vi "Create_column_headers.vi"(1 "ADAM Titles":string[](array[string]), 3 "ADAM Comments":string[](array[string]), 4 "Additional Channels":string[](array[string])) -> (5 "Column headers":string[](array[string]), 6 "Header Comments":string[](array[string]), 7 "No of stats columns":i32[](array[numeric]))   [LabVIEW 2010]
uses:
  Globals/Meas_global.vi
  Globals/Dynamic_call_global.ph.vi
  Globals/LDA_meas_global_1.vi
  Acquisition/PWA/PWAtasksGLOBAL.vi
  Globals/Preference_global.vi
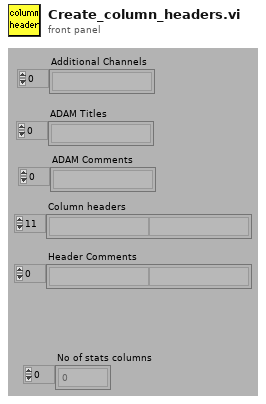
[diagram p1: front panel]
types:
  T1 = typedef "PWA_Data.ctl" = enum16{"No PWA Data", "One Ch PWA"}
  T2 = typedef "Server_Comms.ctl" = enum16{"Server Link Healthy", "Do Not Link To Server"}
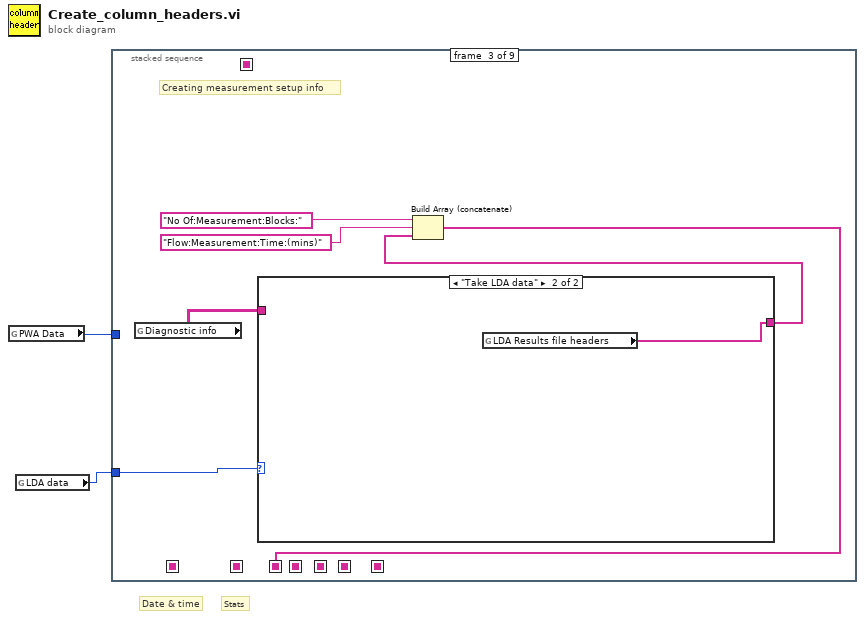
[diagram p0: block diagram]
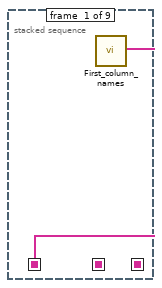
[diagram p2: hidden frame]
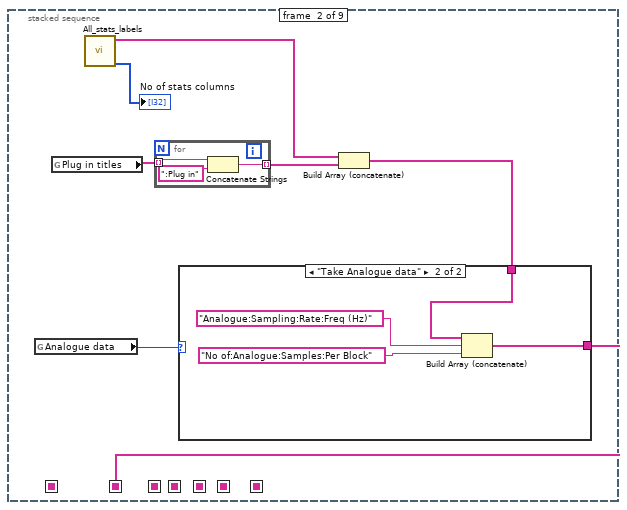
[diagram p3: hidden frame]
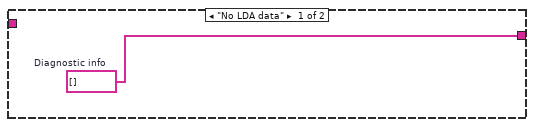
[diagram p5: hidden frame]
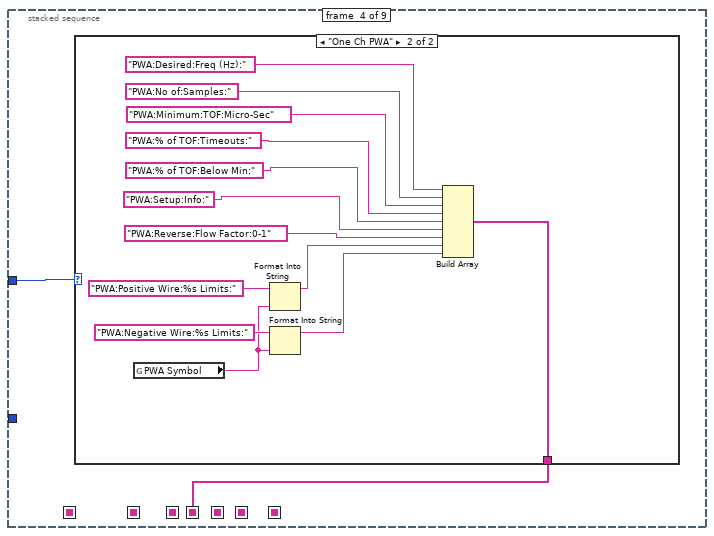
[diagram p6: hidden frame]
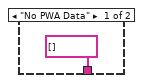
[diagram p7: hidden frame]
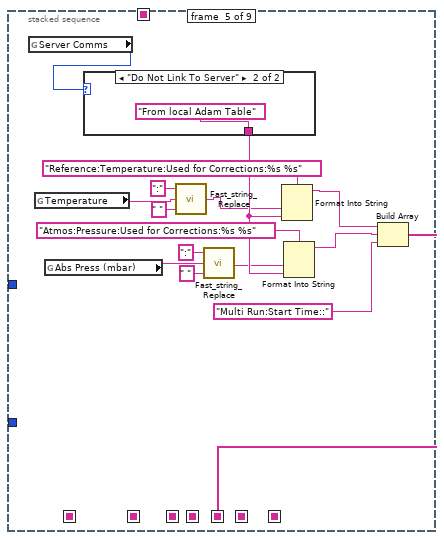
[diagram p8: hidden frame]
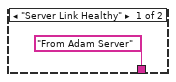
[diagram p9: hidden frame]
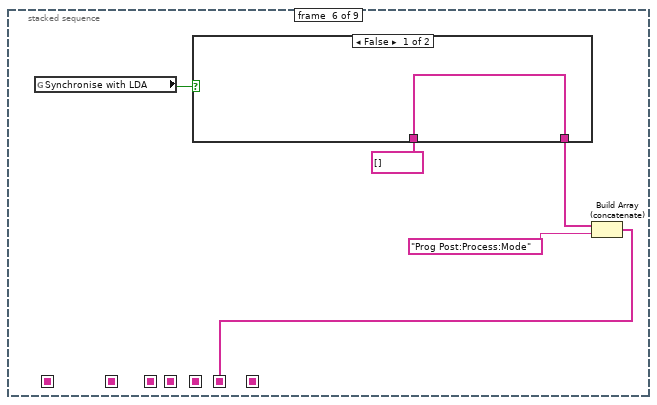
[diagram p10: hidden frame]
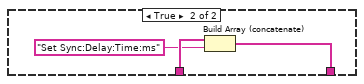
[diagram p11: hidden frame]
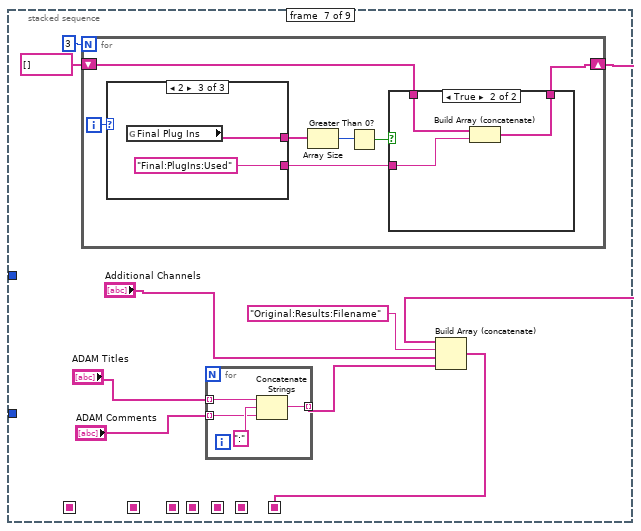
[diagram p12: hidden frame]
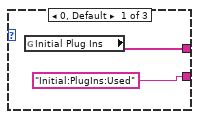
[diagram p14: hidden frame]
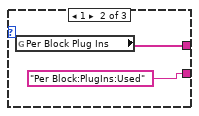
[diagram p15: hidden frame]
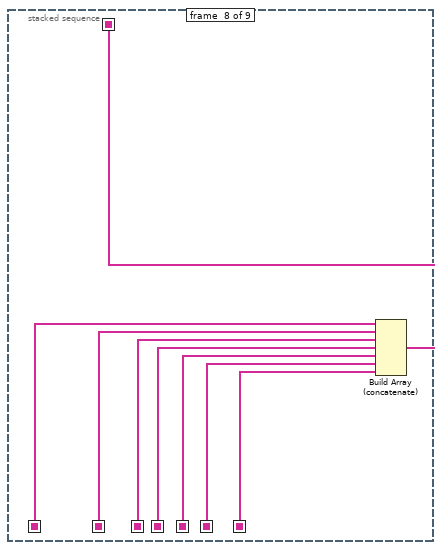
[diagram p16: hidden frame]
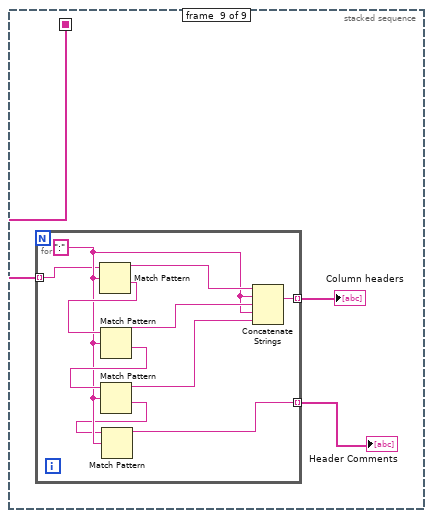
[diagram p17: hidden frame]
diagram:
  # "Stats"
  # "Date & time"
  n1 = global read "Meas_global.vi" "PWA Data"() -> (w1:T1)
  n2 = global read "Meas_global.vi" "LDA data"() -> (w2:enum16{"No LDA data", "Take LDA data"})
  n3 = stacked-sequence {
    seq-local: [_ w4 _ _ _ _ _ _ _] -> [_ _ _ _ _ _ _ w106 _]
    seq-local: [w3 _ _ _ _ _ _ _ _] -> [_ _ _ _ _ _ _ w107 _]
    seq-local: [_ _ w22 _ _ _ _ _ _] -> [_ _ _ _ _ _ _ w105 _]
    seq-local: [_ _ _ _ _ _ w71 _ _] -> [_ _ _ _ _ _ _ w101 _]
    seq-local: [_ _ _ _ w44 _ _ _ _] -> [_ _ _ _ _ _ _ w103 _]
    seq-local: [_ _ _ _ _ _ _ w104 _] -> [_ _ _ _ _ _ _ _ w109]
    seq-local: [_ _ _ _ _ w62 _ _ _] -> [_ _ _ _ _ _ _ w102 _]
    seq-local: [_ _ _ w27 _ _ _ _ _] -> [_ _ _ _ _ _ _ w100 _]
    tunnel: w2 -> [_ _ w20 _ _ _ _ _ _]
    tunnel: w1 -> [_ _ _ w28 _ _ _ _ _]
    frame #0 {
      n4 = call "First_column_names.vi"() -> ("Array"=w3:string[])
    }
    frame #1 {
      n5 = global read "Meas_global.vi" "Analogue data"() -> (w6:enum16{"No Analogue data", "Take Analogue data"})
      n6 = global read "Dynamic_call_global.ph.vi" "Plug in titles"() -> (w9:string[])
      n7 = call "All_stats_labels.vi"() -> ("No of stats columns"=→"No of stats columns":i32[], "Stats labels"=w8:string[])  [unwired: 6 out]
      n8 = for {
        tunnel: w9 -> [w17] mode=indexing
        tunnel: [w18] -> w7 mode=indexing
        n9 = Concatenate Strings(w17, ":Plug in" ("Substring")) -> (w18:string)
      }
      n10 = Build Array (concatenate)(w8, w7) -> (w5:string[])
      n11 = case shown="\"Take Analogue data\"" w6 {
        tunnel: w5 -> [w11 w13]
        tunnel: [w11 w12] -> w4
        frame "No Analogue data" {
        }
        frame "Take Analogue data" {
          n12 = Build Array (concatenate)(w13, "Analogue:Sampling:Rate:Freq (Hz)", "No of:Analogue:Samples:Per Block") -> (w12:string[])
        }
      }
    }
    frame #2 {
      # "Creating measurement setup info"
      n13 = global read "Meas_global.vi" "Diagnostic info"() -> (w21:string[][])
      n14 = case shown="\"Take LDA data\"" w20 {
        tunnel: w21 -> [_ _]
        tunnel: [w25 w26] -> w19
        frame "No LDA data" {
          w25 = string[] []  # Diagnostic info
        }
        frame "Take LDA data" {
          n15 = global read "LDA_meas_global_1.vi" "LDA Results file headers"() -> (w26:string[])
        }
      }
      n16 = Build Array (concatenate)("No Of:Measurement:Blocks:", "Flow:Measurement:Time:(mins)", w19) -> (w22:string[])
    }
    frame #3 {
      n17 = case shown="\"One Ch PWA\"" w28 {
        tunnel: [string[] [] w32] -> w27
        frame "No PWA Data" {
        }
        frame "One Ch PWA" {
          n18 = global read "PWAtasksGLOBAL.vi" "PWA Symbol"() -> (w40:string)
          n19 = Format Into String(format string="PWA:Positive Wire:%s Limits:", w40) -> (resulting string=w34:string)  [unwired: 2 in, 1 out]
          n20 = Format Into String(format string="PWA:Negative Wire:%s Limits:", w40) -> (resulting string=w33:string)  [unwired: 2 in, 1 out]
          n21 = Build Array("PWA:Desired:Freq (Hz):", "PWA:No of:Samples:", "PWA:Minimum:TOF:Micro-Sec", "PWA:% of TOF:Timeouts:", "PWA:% of TOF:Below Min:", "PWA:Setup:Info:", "PWA:Reverse:Flow Factor:0-1", w34, w33) -> (w32:string[])
        }
      }
    }
    frame #4 {
      n22 = global read "Preference_global.vi" "Server Comms"() -> (w58:T2)
      n23 = global read "Preference_global.vi" "Temperature"() -> (w50:string)
      n24 = global read "Preference_global.vi" "Abs Press (mbar)"() -> (w46:string)
      n25 = case shown="\"Do Not Link To Server\"" w58 {
        tunnel: ["From Adam Server" "From local Adam Table"] -> w53
        frame "Server Link Healthy" {
        }
        frame "Do Not Link To Server" {
        }
      }
      n26 = call "Fast_string_Replace.vi"("Replace match with:"=" ", "Input String"=w50, "regular expression"=":") -> ("Output String"=w49:string)  [unwired: 2 out]
      n27 = call "Fast_string_Replace.vi"("Replace match with:"=" ", "Input String"=w46, "regular expression"=":") -> ("Output String"=w45:string)  [unwired: 2 out]
      n28 = Format Into String(format string="Reference:Temperature:Used for Corrections:%s %s", w49, w53) -> (resulting string=w56:string)  [unwired: 2 in, 1 out]
      n29 = Format Into String(format string="Atmos:Pressure:Used for Corrections:%s %s", w45, w53) -> (resulting string=w54:string)  [unwired: 2 in, 1 out]
      n30 = Build Array(w56, w54, "Multi Run:Start Time::") -> (w44:string[])
    }
    frame #5 {
      n31 = global read "Meas_global.vi" "Synchronise with LDA"() -> (w65:bool)
      n32 = case shown="False" w65 {
        tunnel: [w66 w68] -> w63
        tunnel: string[] [] ("Column Titles") -> [w66 w69]
        frame False {
        }
        frame True {
          n33 = Build Array (concatenate)(w69, "Set Sync:Delay:Time:ms" ("Input Element")) -> (w68:string[])
        }
      }
      n34 = Build Array (concatenate)(w63, "Prog Post:Process:Mode" ("Input Element")) -> (w62:string[])
    }
    frame #6 {
      n35 = for {
        N: 3 -> [_]
        shift-right: [w80] -> w72
        shift-left: string[] [] -> [w81]
        i -> [w85]
        n36 = case shown="2" w85 {
          tunnel: [w91 w93 w95] -> w84
          tunnel: ["Initial:PlugIns:Used" ("Input Element") "Per Block:PlugIns:Used" ("Input Element") "Final:PlugIns:Used" ("Input Element")] -> w79
          frame 0, Default {
            n37 = global read "Dynamic_call_global.ph.vi" "Initial Plug Ins"() -> (w91:string[])
          }
          frame 1 {
            n38 = global read "Dynamic_call_global.ph.vi" "Per Block Plug Ins"() -> (w93:string[])
          }
          frame 2 {
            n39 = global read "Dynamic_call_global.ph.vi" "Final Plug Ins"() -> (w95:string[])
          }
        }
        n40 = Array Size(array=w84) -> (size(s)=w83:i32)
        n41 = Greater Than 0?(x=w83) -> (x > 0?=w82:bool)
        n42 = case shown="True" w82 {
          tunnel: w81 -> [w86 w89]
          tunnel: [w86 w88] -> w80
          tunnel: w79 -> [_ w87]
          frame False {
          }
          frame True {
            n43 = Build Array (concatenate)(w89, w87) -> (w88:string[])
          }
        }
      }
      n44 = for {
        tunnel: "ADAM Titles" -> [w98] mode=indexing
        tunnel: "ADAM Comments" -> [w97] mode=indexing
        tunnel: [w96] -> w76 mode=indexing
        n45 = Concatenate Strings(w98, ":" ("Substring"), w97) -> (w96:string)
      }
      n46 = Build Array (concatenate)(w72, "Original:Results:Filename", "Additional Channels", w76) -> (w71:string[])
    }
    frame #7 {
      n47 = Build Array (concatenate)(w107, w106, w105, w100, w103, w102, w101) -> (w104:string[])
    }
    frame #8 {
      n48 = for {
        tunnel: w109 -> [w111] mode=indexing
        tunnel: [w115] -> w108 mode=indexing
        tunnel: [w112] -> w110 mode=indexing
        w114 = ":" ("regular expression")
        n49 = Match Pattern(string=w111, regular expression=w114) -> (before substring=w118:string, after substring=w120:string)  [unwired: 3 out]
        n50 = Match Pattern(string=w120, regular expression=w114) -> (before substring=w117:string, after substring=w119:string)  [unwired: 3 out]
        n51 = Match Pattern(string=w119, regular expression=w114) -> (before substring=w116:string, after substring=w113:string)  [unwired: 3 out]
        n52 = Match Pattern(string=w113, regular expression=w114) -> (before substring=w112:string)  [unwired: 4 out]
        n53 = Concatenate Strings(w118, w114, w117, w114, w116) -> (w115:string)
      }
      "Header Comments" <- w110
      "Column headers" <- w108
    }
  }
